vi "AggregateResults (Image).vi"(7 "Section":string, 8 "error in (no error)":errorcluster, 9 "Image Name":string, 10 "Picture":picture, 11 "Pips in":refnum<class "Pips.lvclass">) -> (0 "error out":errorcluster, 3 "Pips out":refnum<class "Pips.lvclass">)   [LabVIEW 2021, in "Bananas.lvlib" / "Pips.lvclass"]
doc: "Accepts any type.\n\nIf of type Cluster, the Section field defaults to the cluster name. If the cluster name is empty, it will be marked as \"uncategorized\". Each element of the cluster will use the label as the key. If unnamed, they will be labeled element0..elementN-1\n\nIf of any type other than cluster, the Section field must be provided, otherwise it will be marked as \"uncategorized\". The Value label will become the key. If no label is found, it will be skipped."
uses:
  Pips.lvclass
  <vilib>/LabVIEW Open Source Project/Data Manipulation/Variant/OpenVariant.lvlib
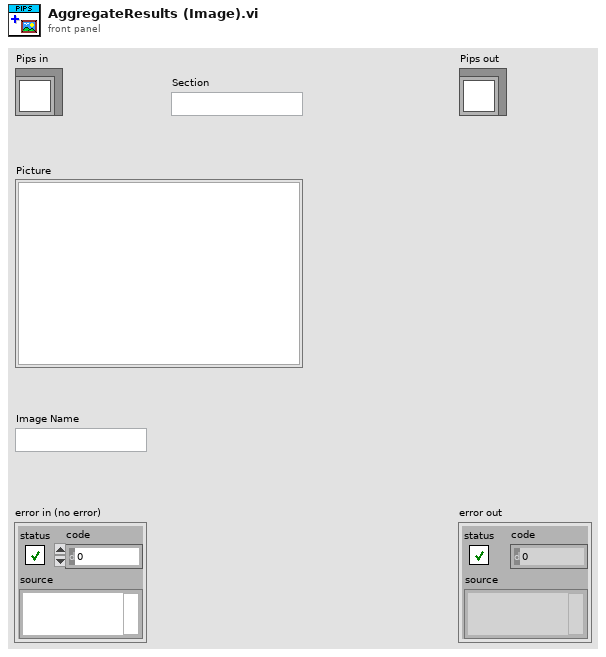
[diagram p1: front panel]
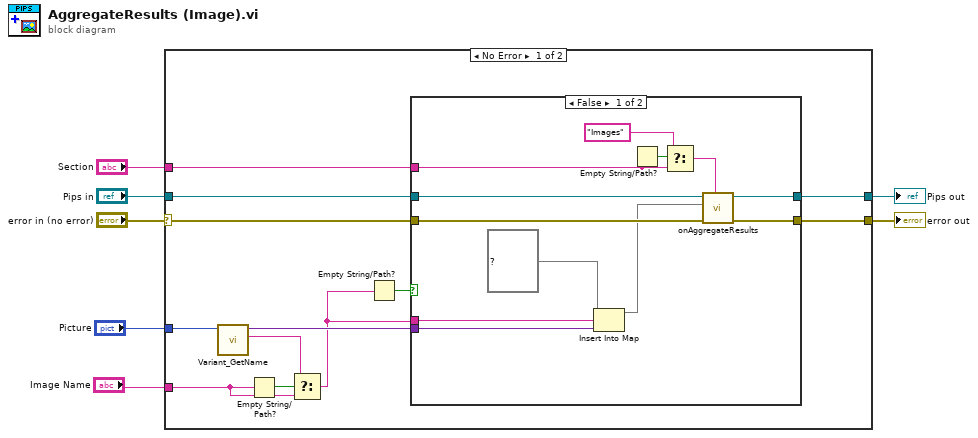
[diagram p0: block diagram]
diagram:
  n1 = case shown="No Error" "error in (no error)" {
    selector: "error in (no error)" -> [w16 w35]
    tunnel: [w17 w35] -> w6
    tunnel: [w18 w34] -> w4
    tunnel: "Pips in" -> [w19 w34]
    tunnel: "Picture" -> [w14 _]
    tunnel: "Section" -> [w15 _]
    tunnel: "Image Name" -> [w10 _]
    frame No Error {
      n2 = call <vilib>:"Variant_GetName.vi"("Variant"=w14) -> ("Name"=w11:string, "Variant dup"=w13:variant)  [unwired: 8 in, 1 out]
      n3 = Empty String/Path?(string/path=w10) -> (empty?=w12:bool)
      n4 = Select(t=w11, s=w12, f=w10) -> (s? t:f=w9:string)
      n5 = Empty String/Path?(string/path=w9) -> (empty?=w8:bool)
      n6 = case shown="False" w8 {
        tunnel: w19 -> [w31 w33]
        tunnel: [w30 w33] -> w18
        tunnel: [w29 w32] -> w17
        tunnel: w16 -> [w28 w32]
        tunnel: w15 -> [w27 _]
        tunnel: w13 -> [w20 _]
        tunnel: w9 -> [w22 _]
        frame False {
          n7 = Insert Into Map(map in=map{string, variant} {} ("Results"), key=w22, value=w20) -> (map out=w25:map{string, variant})  [unwired: 2 out]
          n8 = Empty String/Path?(string/path=w27) -> (empty?=w24:bool)
          n9 = Select(t="Images", s=w24, f=w27) -> (s? t:f=w26:string)
          n10 = call-dynamic "onAggregateResults.vi"("Section"=w26, "error in (no error)"=w28, "Results"=w25, "Pips in"=w31) -> ("error out"=w29:errorcluster, "Pips out"=w30:refnum<class "Pips.lvclass">)  [unwired: 6 in]
        }
        frame True {
        }
      }
    }
    frame Error {
    }
  }
  "error out" <- w6
  "Pips out" <- w4
